vi "ElapsedTimeCounter.vi"(8 "Error In":errorcluster, 9 "Dwell Time (seconds)":dbl, 10 "InitialMillisecondTimerValue":dbl, 11 "Elapsed Seconds (In)":dbl) -> (0 "Error Out":errorcluster, 2 "Minimum Dwell Met?":bool, 3 "Elapsed Seconds (Out)":dbl)   [LabVIEW 2020]
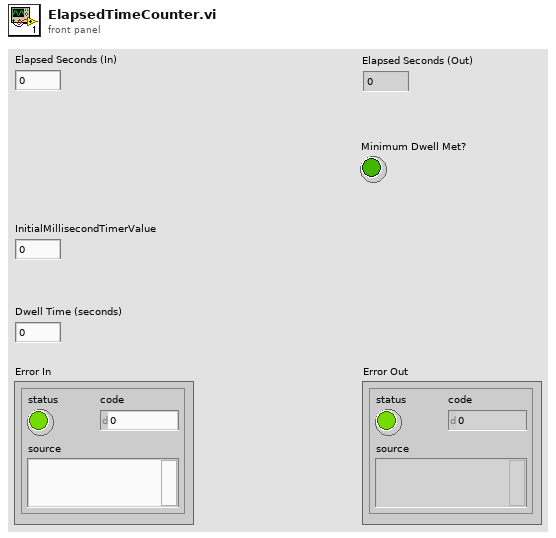
[diagram p1: front panel]
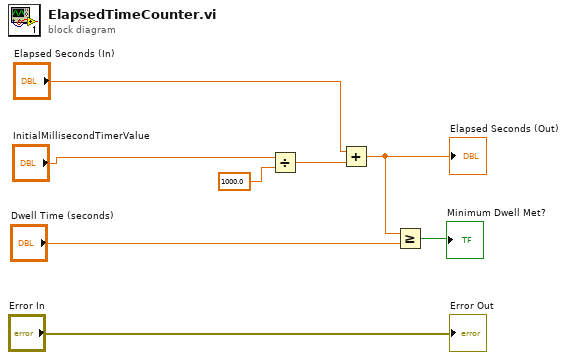
[diagram p0: block diagram]
diagram:
  n1 = Divide(x="InitialMillisecondTimerValue", y=1000.0) -> (x/y=w3:dbl)
  n2 = Add(x="Elapsed Seconds (In)", y=w3) -> (x+y=w6:dbl)
  "Elapsed Seconds (Out)" <- w6
  n3 = Greater Or Equal?(x=w6, y="Dwell Time (seconds)") -> (x >= y?=→"Minimum Dwell Met?":bool)
  "Error Out" <- "Error In"
